vi "Write Data.vi"(8 "error in (no error)":errorcluster, 10 "Data":string, 11 "TCP Stream in":refnum<class "TCP Stream.lvclass">) -> (0 "error out":errorcluster, 3 "TCP Stream out":refnum<class "TCP Stream.lvclass">)   [LabVIEW 2020, in "Stream-TCP.lvlib" / "TCP Stream.lvclass"]
uses:
  TCP Stream.lvclass
  TCP Stream.lvclass/TCP Stream.ctl
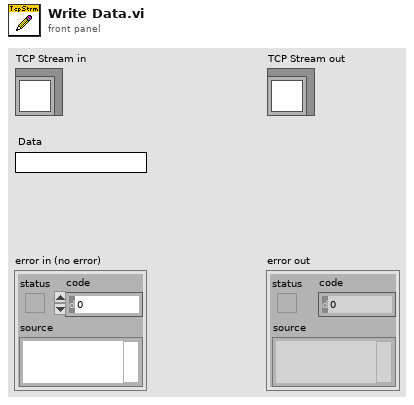
[diagram p1: front panel]
types:
  T1 = enum16{"Standard", "Buffered", "CRLF", "Immediate"}
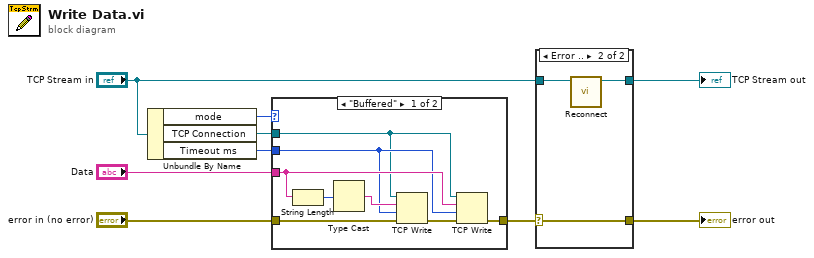
[diagram p0: block diagram]
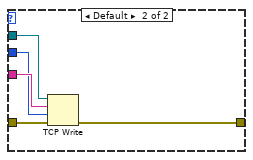
[diagram p2: hidden frame]
diagram:
  n1 = Unbundle By Name("TCP Stream in") -> ("mode"=w4:T1, "TCP Connection"=w9:refnum<k5>, "Timeout ms"=w3:i32)
  n2 = case shown="\"Buffered\"" w4 {
    tunnel: "error in (no error)" -> [w17 w22]
    tunnel: w9 -> [w11 w21]
    tunnel: "Data" -> [w13 w20]
    tunnel: [w10 w19] -> w7
    tunnel: w3 -> [w12 w18]
    frame "Buffered" {
      n3 = String Length(string=w13) -> (length=w16:i32)
      n4 = Type Cast(x=w16) -> (*(type *) &x=w15:string)  [unwired: 1 in]
      n5 = TCP Write(connection ID=w11, data in=w15, error in (no error)=w17, 9:w12) -> (error out=w14:errorcluster)  [unwired: 2 out]
      n6 = TCP Write(connection ID=w11, data in=w13, error in (no error)=w14, 9:w12) -> (error out=w10:errorcluster)  [unwired: 2 out]
    }
    frame Default {
      n7 = TCP Write(connection ID=w21, data in=w20, error in (no error)=w22, 9:w18) -> (error out=w19:errorcluster)  [unwired: 2 out]
    }
  }
  n8 = case shown="Error .." w7 {
    selector: w7 -> [w23 w26]
    tunnel: "TCP Stream in" -> [w24 w27]
    tunnel: [w23 w26] -> w1
    tunnel: [w24 w25] -> w5
    frame No Error {
    }
    frame Error {
      n9 = call "Reconnect.vi"("TCP Stream in"=w27) -> ("TCP Stream out"=w25:refnum<class "TCP Stream.lvclass">)  [unwired: 9 in, 1 out]
    }
  }
  "error out" <- w1
  "TCP Stream out" <- w5
